vi "Utility_Main.vi"() -> ()   [LabVIEW 2017, in "GL860_Driver.lvlib"]
uses:
  GL860_Driver.lvlib
panel:
  in  "Path":string="MEM\\" caption="ファイル選択"
  in  "CSV_Convert":bool
  in  "File_List":bool
  in  "Digital_Monitor":bool
  in  "Graph Monitor":bool
  in  "Recording":bool
  in  "UDP_Connect":bool
  in  "CommandLine":bool
  out "Connect?":bool
  in  "接続":bool
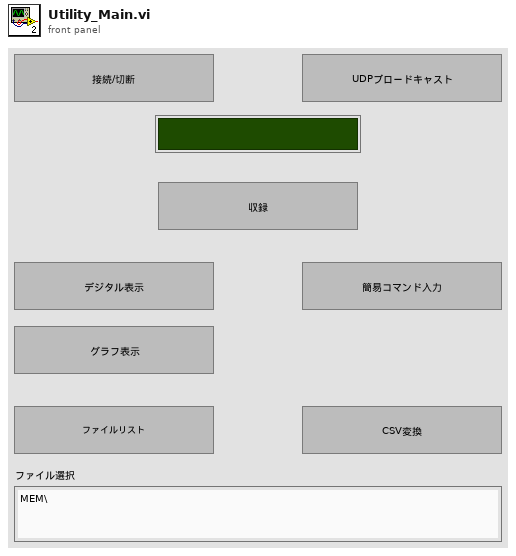
[diagram p1: front panel]
types:
  T1 = typedef "ConnectionID.ctl" = cluster{"Mode":enum16{"TCP/IP", "USB"}, "TCP/IP":refnum<k5>, "USB":i32}
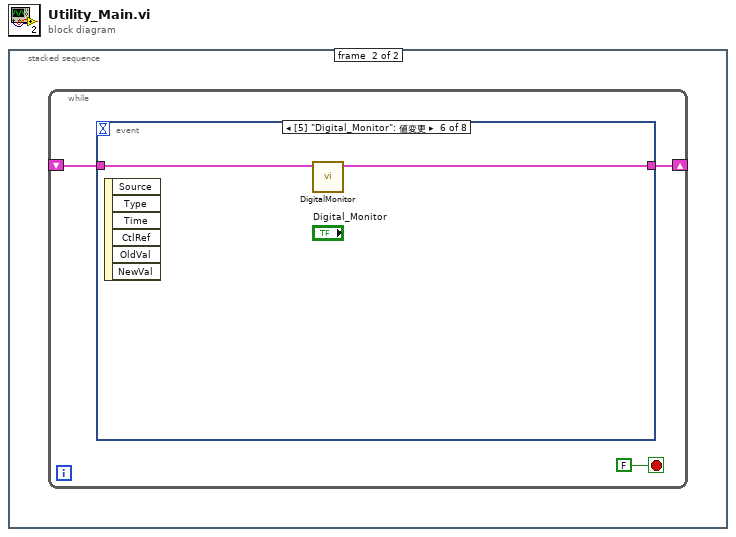
[diagram p0: block diagram]
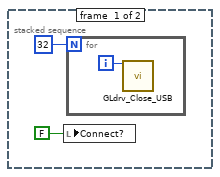
[diagram p2: hidden frame]
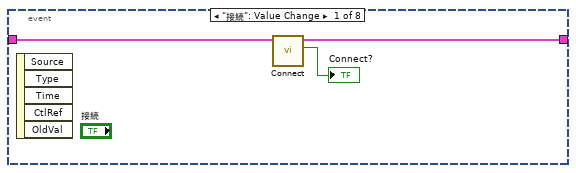
[diagram p3: hidden frame]
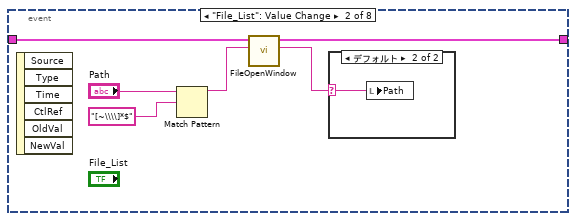
[diagram p4: hidden frame]
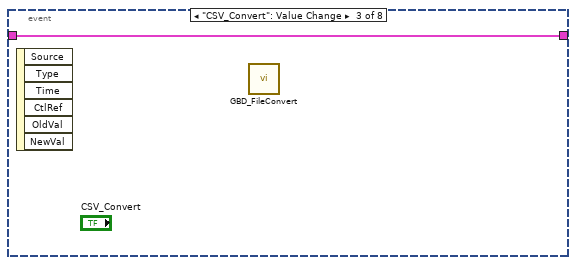
[diagram p6: hidden frame]
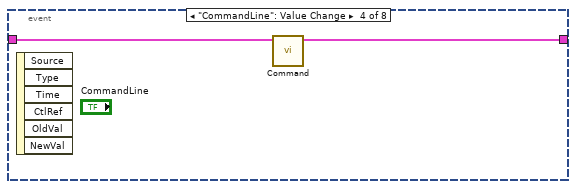
[diagram p7: hidden frame]
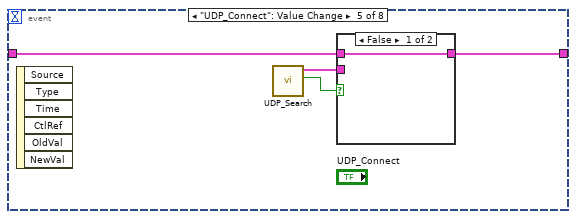
[diagram p8: hidden frame]
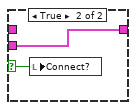
[diagram p9: hidden frame]
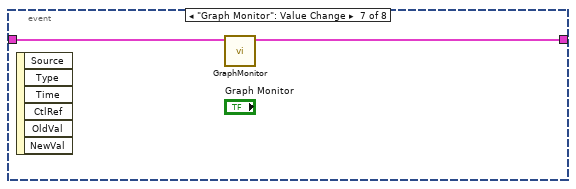
[diagram p10: hidden frame]
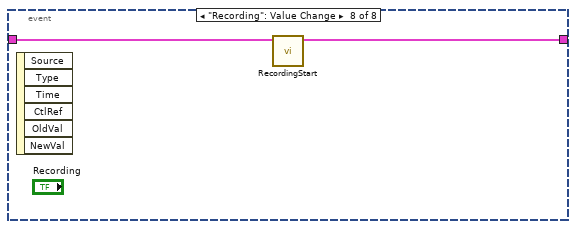
[diagram p11: hidden frame]
diagram:
  n1 = stacked-sequence {
    frame #0 {
      n2 = local write "Connect?"(FALSE ("Connect?")) -> ()
      n3 = for {
        N: 32 -> [_]
        i -> [w3]
        n4 = call "GLdrv_Close_USB.vi"("hDevice"=w3) -> ()  [unwired: 1 in, 14 out]
      }
    }
    frame #1 {
      n5 = while {
        shift-right: [w6] -> _
        shift-left: _ -> [w5]
        stop <- FALSE stop-if-true
        n6 = event shown="[5] \"Digital_Monitor\": 値変更" {
          selector: _ -> [_ _ _ _ _ _ _ _]
          dyn-events: _ -> [_ _ _ _ _ _ _ _]
          timeout: _ -> [_ _ _ _ _ _ _ _]
          tunnel: [w9 w14 w17 w18 w21 w27 w29 w31] -> w6
          tunnel: w5 -> [w8 w15 w17 w19 w20 w28 w30 w32]
          event "接続": Value Change {
            n7 = event-data() -> ()  [unwired: 1 in, 5 out]
            n8 = call "Connect.vi"("Connection ID"=w8) -> ("Connect?"=→"Connect?":bool, "Connection ID Out"=w9:T1)  [unwired: 9 in]
          }
          event "File_List": Value Change {
            n9 = event-data() -> ()  [unwired: 1 in, 6 out]
            n10 = Match Pattern(string="Path", regular expression="[~\\\\]*$") -> (before substring=w11:string)  [unwired: 1 in, 3 out]
            n11 = call "FileOpenWindow.vi"("Path In"=w11, "Connection ID"=w15) -> ("Path Out"=w13:string, "Connection ID Out"=w14:T1)  [unwired: 7 in, 1 out]
            n12 = case shown="デフォルト" w13 {
              selector: w13 -> [_ w16]
              frame "" {
              }
              frame Default {
                n13 = local write "Path"(w16) -> ()
              }
            }
          }
          event "CSV_Convert": Value Change {
            n14 = event-data() -> ()  [unwired: 1 in, 6 out]
            n15 = call "GBD_FileConvert.vi"() -> ()  [unwired: 12 in]
          }
          event "CommandLine": Value Change {
            n16 = event-data() -> ()  [unwired: 1 in, 6 out]
            n17 = call "Command.vi"("Connection ID"=w19) -> ("Connection ID Out"=w18:T1)  [unwired: 10 in]
          }
          event "UDP_Connect": Value Change {
            n18 = event-data() -> ()  [unwired: 1 in, 6 out]
            n19 = call "UDP_Search.vi"() -> ("Connect?"=w23:bool, "Connection ID Out"=w22:T1)  [unwired: 10 in]
            n20 = case shown="FALSE" w23 {
              selector: w23 -> [_ w26]
              tunnel: w22 -> [_ w25]
              tunnel: [w24 w25] -> w21
              tunnel: w20 -> [w24 _]
              frame False {
              }
              frame True {
                n21 = local write "Connect?"(w26) -> ()
              }
            }
          }
          event "Digital_Monitor": Value Change {
            n22 = event-data() -> ()  [unwired: 1 in, 6 out]
            n23 = call "DigitalMonitor.vi"("Connection ID"=w28) -> ("Connection ID Out"=w27:T1)  [unwired: 9 in, 1 out]
          }
          event "Graph Monitor": Value Change {
            n24 = event-data() -> ()  [unwired: 1 in, 6 out]
            n25 = call "GraphMonitor.vi"("Connection ID"=w30) -> ("Connection ID Out"=w29:T1)  [unwired: 9 in, 1 out]
          }
          event "Recording": Value Change {
            n26 = event-data() -> ()  [unwired: 1 in, 6 out]
            n27 = call "RecordingStart.vi"("Connection ID"=w32) -> ("Connection ID Out"=w31:T1)  [unwired: 10 in]
          }
        }
      }
    }
  }
